vi "Main.vi"() -> ()   [LabVIEW 2017]
doc: "The myRIO Project template acquires acceleration data from the onboard accelerometer and displays the changes of acceleration values in a waveform chart."
uses:
  <vilib>/myRIO/Common/Instrument Driver Framework/myRIO v1.0/UART/vis/myRIO v1.0 Close UART.vi
  <vilib>/myRIO/Common/Instrument Driver Framework/Utilities/vis/FPGA Ref Manager.vi
  <vilib>/myRIO/Common/Instrument Driver Framework/myRIO v1.0/myRIO v1.0 Reset FPGA.vi
  <vilib>/myRIO/Common/Instrument Driver Framework/myRIO v1.0/IRQ/vis/myRIO v1.0 IRQ Info FGV.vi
  <vilib>/myRIO/Common/Instrument Driver Framework/myRIO v1.0/IRQ/vis/myRIO v1.0 Timer IRQ Info FGV.vi
  <vilib>/myRIO/Common/Instrument Driver Framework/myRIO v1.0/IRQ/vis/myRIO v1.0 ISR Agent.vi
  <vilib>/myRIO/Instrument Drivers/Utilities/Utilities.lvlib
panel:
  out "error out":errorcluster
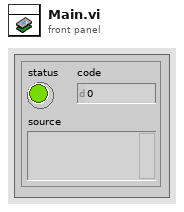
[diagram p1: front panel]
types:
  T1 = enum16{"Terminate", "Finalize", "Execute", "Initialize"}
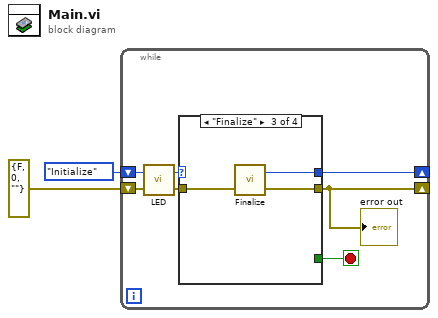
[diagram p0: block diagram]
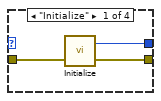
[diagram p2: hidden frame]
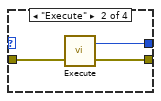
[diagram p3: hidden frame]
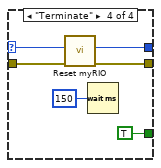
[diagram p4: hidden frame]
diagram:
  n1 = while {
    shift-right: [w8] -> _
    shift-left: errorcluster {"status"=FALSE, "code"=0, "source"=""} ("error in (no error)") -> [w5]
    shift-right: [w6] -> _
    shift-left: T1."Initialize" -> [w3]
    stop <- w7 stop-if-true
    n2 = call "LED.vi"("error in (no error)"=w5, "Enum"=w3) -> ("error out"=w4:errorcluster)  [unwired: 1 in]
    n3 = case shown="\"Finalize\"" w3 {
      selector: w3 -> [_ _ _ w19]
      tunnel: [w10 w13 w16 w21] -> w8
      tunnel: [w9 w12 w15 w19] -> w6
      tunnel: w4 -> [w11 w14 w17 w22]
      tunnel: [_ _ _ TRUE] -> w7
      frame "Initialize" {
        n4 = call "Initialize.vi"("error in"=w11) -> ("error out"=w10:errorcluster, "Enum"=w9:T1)  [unwired: 1 in]
      }
      frame "Execute" {
        n5 = call "Execute.vi"("error in"=w14) -> ("error out"=w13:errorcluster, "Enum"=w12:T1)  [unwired: 1 in]
      }
      frame "Finalize" {
        n6 = call "Finalize.vi"("error in (no error)"=w17) -> ("error out"=w16:errorcluster, "Enum"=w15:T1)  [unwired: 1 in]
      }
      frame "Terminate" {
        n7 = call <vilib>:"Reset myRIO.vi"("error in (no error)"=w22) -> ("error out"=w21:errorcluster)  [unwired: 10 in]
        n8 = Wait (ms)(milliseconds to wait=u32 150) -> ()  [unwired: 1 out]
      }
    }
    "error out" <- w8
  }
